vi "Is Error Selected.vi"(7 "global scope?":T1=enum."global", 8 "error in (no error)":errorcluster, 10 "selected error":T2, 11 "error codes files":variant) -> (0 "error out":errorcluster, 2 "editable?":bool, 3 "selected?":bool)   [LabVIEW 2017]
uses:
  Error List/Error Owner and ID.ctl
  Error List/Scope.ctl
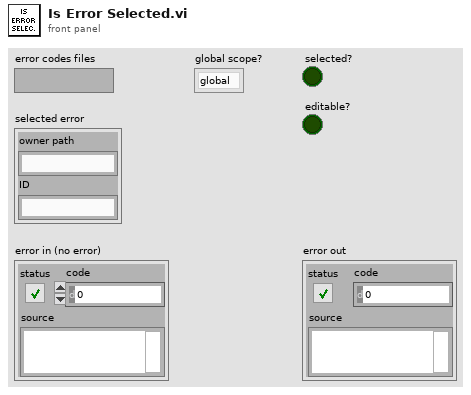
[diagram p1: front panel]
types:
  T1 = typedef "Scope.ctl" = enum16{"project", "global"}
  T2 = typedef "Error Owner and ID.ctl" = cluster{"owner path":string, "ID":string}
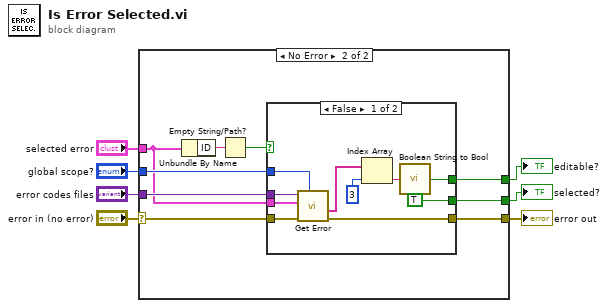
[diagram p0: block diagram]
diagram:
  n1 = case shown="No Error" "error in (no error)" {
    selector: "error in (no error)" -> [w8 w17]
    tunnel: "selected error" -> [_ w13]
    tunnel: "global scope?" -> [_ w14]
    tunnel: "error codes files" -> [_ w15]
    tunnel: [w8 w11] -> w3
    tunnel: [_ w10] -> w2
    tunnel: [_ w9] -> w1
    frame Error {
    }
    frame No Error {
      n2 = Unbundle By Name(w13) -> ("ID"=w16:string)
      n3 = Empty String/Path?(string/path=w16) -> (empty?=w12:bool)
      n4 = case shown="False" w12 {
        tunnel: [w27 w28] -> w11
        tunnel: w17 -> [w26 w28]
        tunnel: w15 -> [w25 _]
        tunnel: w14 -> [w24 _]
        tunnel: w13 -> [w23 _]
        tunnel: [TRUE _] -> w10
        tunnel: [w19 _] -> w9
        frame False {
          n5 = call "Get Error.vi"("scope"=w24, "error in (no error)"=w26, "owner error"=w23, "error list <top>"=w25) -> ("error out"=w27:errorcluster, "attributes"=w18:string[])  [unwired: 3 in, 3 out]
          n6 = Index Array(array=w18, index=3) -> (element=w21:string)
          n7 = call "Boolean String to Bool.vi"("boolean string"=w21) -> ("true?"=w19:bool)
        }
        frame True {
        }
      }
    }
  }
  "error out" <- w3
  "editable?" <- w1
  "selected?" <- w2
